vi "Write bev.vi"(8 "error in (no error)":errorcluster, 10 "Beverage.lvclass":refnum<class "Beverage.lvclass">, 11 "CondimentDecorator in":refnum<class "CondimentDecorator.lvclass">) -> (0 "error out":errorcluster, 3 "CondimentDecorator out":refnum<class "CondimentDecorator.lvclass">)   [LabVIEW 2017, in "CondimentDecorator.lvclass"]
uses:
  CondimentDecorator.lvclass
  Beverage Class/Beverage.lvclass
  CondimentDecorator.lvclass/CondimentDecorator.ctl
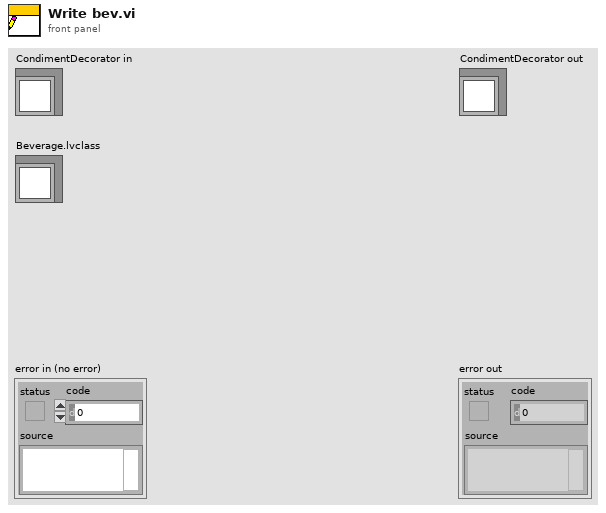
[diagram p1: front panel]
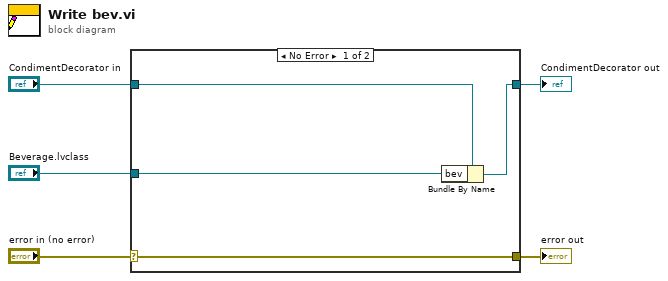
[diagram p0: block diagram]
diagram:
  n1 = case shown="No Error" "error in (no error)" {
    selector: "error in (no error)" -> [w9 w10]
    tunnel: [w9 w10] -> w4
    tunnel: [w7 w11] -> w2
    tunnel: "CondimentDecorator in" -> [w8 w11]
    tunnel: "Beverage.lvclass" -> [w6 _]
    frame No Error {
      n2 = Bundle By Name(cluster=w8, "bev"=w6) -> (w7:refnum<class "CondimentDecorator.lvclass">)
    }
    frame Error {
    }
  }
  "error out" <- w4
  "CondimentDecorator out" <- w2
